vi "Actuation GUI - 030522.vi"() -> ()   [LabVIEW 2021]
uses:
  <vilib>/numeric/Random Number (Range) DBL.vi
panel:
  in  "Duty Cycle":i16(knob) scale=0.0..100.0
  in  "Load Torque":dbl(knob) scale=-0.2..0.2
  in  "Data Update Speed (ms)":u32
  out "Single Plot (Array of X,Y Pairs) 3":cluster{i32, dbl}[](graph)
  out "Single Plot (Array of X,Y Pairs) 2":cluster{i32, dbl}[](graph)
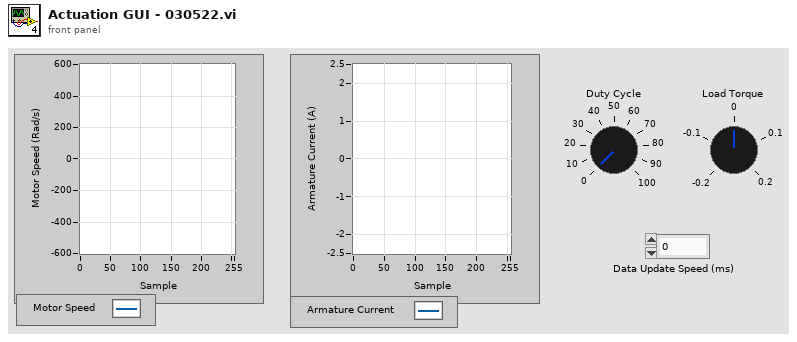
[diagram p1: front panel]
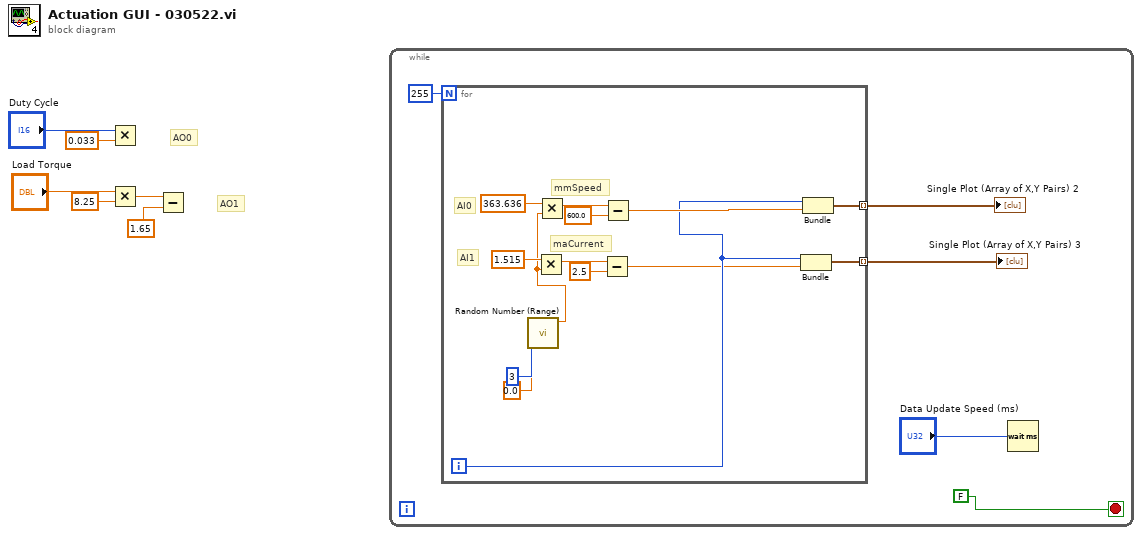
[diagram p0: block diagram]
diagram:
  # "AO1"
  # "AO0"
  n1 = Multiply(x="Duty Cycle", y=0.033) -> ()  [unwired: 1 out]
  n2 = Multiply(x="Load Torque", y=8.25) -> (x*y=w2:dbl)
  n3 = Subtract(x=w2, y=1.65) -> ()  [unwired: 1 out]
  n4 = while {
    stop <- FALSE ("stop") stop-if-true
    n5 = for {
      N: 255 -> [_]
      tunnel: [w19] -> w11 mode=indexing
      tunnel: [w18] -> w10 mode=indexing
      i -> [w16]
      # "AI1"
      # "AI0"
      # "maCurrent"
      # "mmSpeed"
      n6 = call-poly <vilib>:"Random Number (Range).vi"("lower bound (0)"=0.0, "upper bound (100)"=u64 3) -> ("number"=w12:dbl)  [unwired: 9 in]
      n7 = Multiply(x=1.515, y=w12) -> (x*y=w25:dbl)
      n8 = Multiply(x=363.636, y=w12) -> (x*y=w24:dbl)
      n9 = Subtract(x=w25, y=2.5) -> (x-y=w15:dbl)
      n10 = Subtract(x=w24, y=600.0) -> (x-y=w17:dbl)
      n11 = Bundle(w16, w15) -> (w18:cluster{i32, dbl})  [unwired: 1 in]
      n12 = Bundle(w16, w17) -> (w19:cluster{i32, dbl})  [unwired: 1 in]
    }
    "Single Plot (Array of X,Y Pairs) 2" <- w11
    "Single Plot (Array of X,Y Pairs) 3" <- w10
    n13 = Wait (ms)(milliseconds to wait="Data Update Speed (ms)") -> ()  [unwired: 1 out]
  }
